vi "End Game.vi"(11 "MyTeam in":refnum<class "MyTeam.lvclass">) -> (3 "MyTeam out":refnum<class "MyTeam.lvclass">)   [LabVIEW 2020, in "SquareTeam.lvlib" / "MyTeam.lvclass"]
uses:
  MyTeam.lvclass
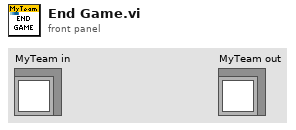
[diagram p1: front panel]
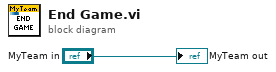
[diagram p0: block diagram]
diagram:
  "MyTeam out" <- "MyTeam in"
